vi "KepcoDCPwr Measure [MSR].vi"(0 "VISA Session":refnum<visa-resource-name>, 1 "Virtual Voltage":dbl format="%.2f", 2 "Virtual Current":dbl format="%.2f", 3 "Virtual Resistance":dbl format="%.2f", 5 "Model In":string, 7 "channel name (\"1\")":string="\"1\"", 9 "measurement type (voltage)":enum16{"Voltage", "Current"}(ring), 11 "error in (no error)":errorcluster {"code" format="%.0x"}) -> (4 "VISA Session Out":refnum<visa-resource-name>, 6 "Model Out":string, 8 "channel name out (\"\")":string="\"\"" caption="channel name Out (\"\")", 10 "measurement":dbl format="%^.2e", 15 "error out":errorcluster {"code" format="%.0x"})   [LabVIEW 2013]
doc: "This VI takes a measurement on the output signal and returns the measured value."
uses:
  Match Regular Expression.xnode
panel:
  out "return count":u32
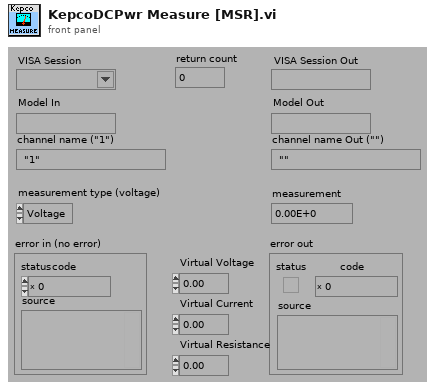
[diagram p1: front panel]
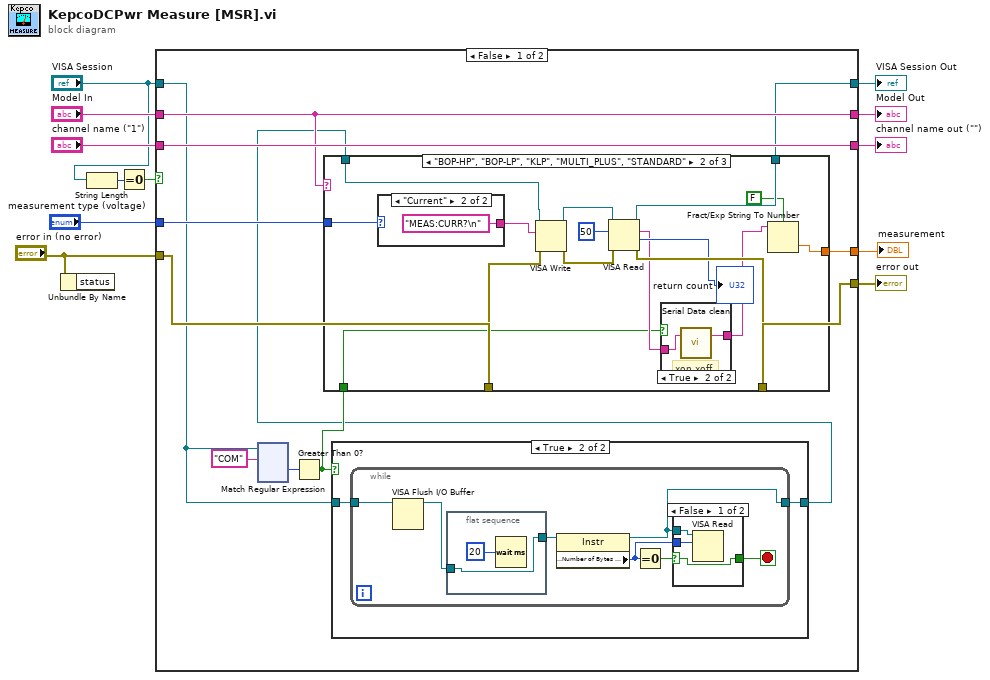
[diagram p0: block diagram]
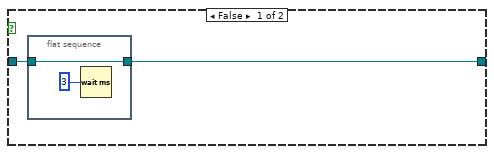
[diagram p2: hidden frame]
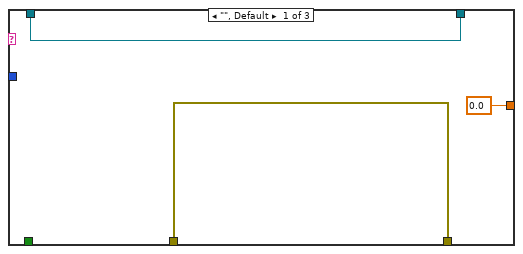
[diagram p4: hidden frame]
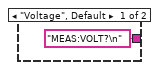
[diagram p6: hidden frame]
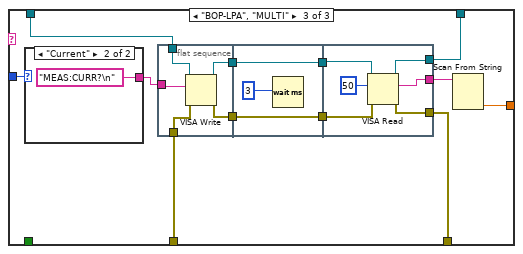
[diagram p7: hidden frame]
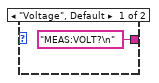
[diagram p8: hidden frame]
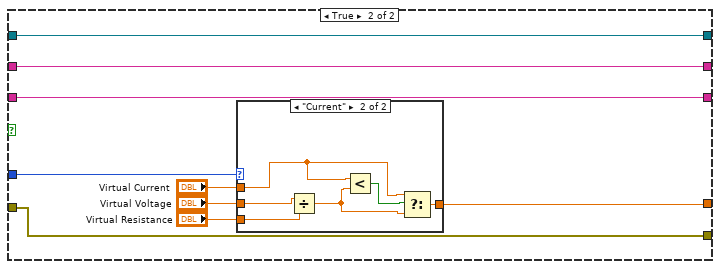
[diagram p9: hidden frame]
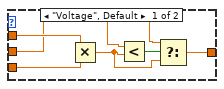
[diagram p10: hidden frame]
diagram:
  n1 = Unbundle By Name("error in (no error)") -> ()  [unwired: 1 out]
  n2 = String Length(string="VISA Session") -> (length=w3:i32)
  n3 = Equal To 0?(x=w3) -> (x = 0?=w2:bool)
  n4 = case shown="False" w2 {
    tunnel: [w22 w214] -> w12
    tunnel: "error in (no error)" -> [w21 w214]
    tunnel: "VISA Session" -> [w13 w213]
    tunnel: "Model In" -> [w23 w212]
    tunnel: "channel name (\"1\")" -> [w24 w211]
    tunnel: [w20 w213] -> w8
    tunnel: [w23 w212] -> w7
    tunnel: [w24 w211] -> w6
    tunnel: [w19 w206] -> w5
    tunnel: "measurement type (voltage)" -> [w18 w210]
    frame False {
      n5 = xnode "Match Regular Expression"("input string"=w13, "regular expression"="COM") -> ("offset past match"=w16:i32)  [unwired: 2 in, 6 out]
      n6 = Greater Than 0?(x=w16) -> (x > 0?=w15:bool)
      n7 = case shown="True" w15 {
        tunnel: [w26 w30] -> w14
        tunnel: w13 -> [w25 w29]
        frame False {
          n8 = flat-sequence {
            tunnel: w25 -> [w28]
            tunnel: [w28] -> w26
            frame #0 {
              n9 = Wait (ms)(milliseconds to wait=u32 3 ("byte count (0)")) -> ()  [unwired: 1 out]
            }
          }
        }
        frame True {
          n10 = while {
            tunnel: w29 -> [w33]
            tunnel: [w35] -> w30
            stop <- w36 stop-if-true
            n11 = VISA Flush I/O Buffer(VISA resource name=w33) -> (VISA resource name out=w32:refnum<visa-resource-name>)  [unwired: 2 in, 1 out]
            n12 = flat-sequence {
              tunnel: w32 -> [w38]
              tunnel: [w38] -> w31
              frame #0 {
                n13 = Wait (ms)(milliseconds to wait=u32 20) -> ()  [unwired: 1 out]
              }
            }
            n14 = property class="Instr"(reference=w31) -> (reference out=w35:refnum<visa-resource-name>, "Serial Settings:Number of Bytes at Serial Port"=w34:u32)  [unwired: 1 in, 1 out]
            n15 = Equal To 0?(x=w34) -> (x = 0?=w37:bool)
            n16 = case shown="False" w37 {
              selector: w37 -> [w42 w43]
              tunnel: [w42 w43] -> w36
              tunnel: w35 -> [w41 _]
              tunnel: w34 -> [w40 _]
              frame False {
                n17 = VISA Read(VISA resource name=w41, byte count=w40) -> ()  [unwired: 1 in, 4 out]
              }
              frame True {
              }
            }
          }
        }
      }
      n18 = case shown="\"BOP-HP\", \"BOP-LP\", \"KLP\", \"MULTI_PLUS\", \"STANDARD\"" w23 {
        tunnel: [w155 w165 w180] -> w20
        tunnel: w14 -> [w155 w170 w187]
        tunnel: w18 -> [_ w171 w188]
        tunnel: w21 -> [w157 w169 w186]
        tunnel: [w157 w164 w179] -> w22
        tunnel: [0.0 w168 w185] -> w19
        tunnel: w15 -> [_ w158 _]
        frame "", Default {
        }
        frame "BOP-HP", "BOP-LP", "KLP", "MULTI_PLUS", "STANDARD" {
          n19 = case shown="\"Current\"" w171 {
            tunnel: ["MEAS:VOLT?\n" "MEAS:CURR?\n"] -> w172
            frame "Voltage", Default {
            }
            frame "Current" {
            }
          }
          n20 = VISA Write(VISA resource name=w170, write buffer=w172, error in (no error)=w169) -> (VISA resource name out=w166:refnum<visa-resource-name>, error out=w167:errorcluster)  [unwired: 1 out]
          n21 = VISA Read(VISA resource name=w166, byte count=u32 50 ("byte count (0)"), error in (no error)=w167) -> (VISA resource name out=w165:refnum<visa-resource-name>, read buffer=w160:string, return count=→"return count":u32, error out=w164:errorcluster)
          n22 = case shown="True" w158 {
            tunnel: [w173 w174] -> w159
            tunnel: w160 -> [w173 w175]
            frame False {
            }
            frame True {
              # "xon xoff"
              n23 = call "Serial Data clean.vi"("string"=w175) -> ("Stripped of Xon Xoff"=w174:string)  [unwired: 2 in]
            }
          }
          n24 = Fract/Exp String To Number(use system decimal point (T)=FALSE, string=w159) -> (number=w168:dbl)  [unwired: 2 in, 1 out]
        }
        frame "BOP-LPA", "MULTI" {
          n25 = case shown="\"Current\"" w188 {
            tunnel: ["MEAS:VOLT?\n" "MEAS:CURR?\n"] -> w189
            frame "Voltage", Default {
            }
            frame "Current" {
            }
          }
          n26 = flat-sequence {
            tunnel: w189 -> [w194]
            tunnel: w187 -> [w193]
            tunnel: w186 -> [w192]
            tunnel: [w191] -> w184
            tunnel: [w190] -> w183
            tunnel: w184 -> [w197]
            tunnel: w183 -> [w196]
            tunnel: [w197] -> w182
            tunnel: [w196] -> w181
            tunnel: [w199] -> w180
            tunnel: [w200] -> w179
            tunnel: w182 -> [w202]
            tunnel: w181 -> [w201]
            tunnel: [w198] -> w178
            frame #0 {
              n27 = VISA Write(VISA resource name=w193, write buffer=w194, error in (no error)=w192) -> (VISA resource name out=w190:refnum<visa-resource-name>, error out=w191:errorcluster)  [unwired: 1 out]
            }
            frame #1 {
              n28 = Wait (ms)(milliseconds to wait=3) -> ()  [unwired: 1 out]
            }
            frame #2 {
              n29 = VISA Read(VISA resource name=w201, byte count=u32 50 ("byte count (0)"), error in (no error)=w202) -> (VISA resource name out=w199:refnum<visa-resource-name>, read buffer=w198:string, error out=w200:errorcluster)  [unwired: 1 out]
            }
          }
          n30 = Scan From String(input string=w178) -> (output 1=w185:dbl)  [unwired: 3 in, 4 out]
        }
      }
    }
    frame True {
      n31 = case shown="\"Current\"" w210 {
        tunnel: "Virtual Current" -> [w220 w221]
        tunnel: "Virtual Voltage" -> [w215 w225]
        tunnel: "Virtual Resistance" -> [w219 w226]
        tunnel: [w218 w224] -> w206
        frame "Voltage", Default {
          n32 = Multiply(x=w220, y=w219) -> (x*y=w216:dbl)
          n33 = Less?(x=w215, y=w216) -> (x < y?=w217:bool)
          n34 = Select(t=w215, s=w217, f=w216) -> (s? t:f=w218:dbl)
        }
        frame "Current" {
          n35 = Divide(x=w225, y=w226) -> (x/y=w223:dbl)
          n36 = Less?(x=w221, y=w223) -> (x < y?=w222:bool)
          n37 = Select(t=w221, s=w222, f=w223) -> (s? t:f=w224:dbl)
        }
      }
    }
  }
  "error out" <- w12
  "channel name out (\"\")" <- w6
  "Model Out" <- w7
  "VISA Session Out" <- w8
  "measurement" <- w5
